vi "Eigenschaften laden.vi"(8 "error in (no error)":errorcluster caption="Fehler (Eingang)", 11 "TDMS-Datei":refnum<k34>) -> (0 "error out":errorcluster caption="Fehler (Ausgang)", 1 "Datentypen":string[](array[string]), 2 "Namen":string[](array[string]), 3 "TDMS-Datei (Ausgang)":refnum<k34>, 4 "Eigenschaften":T1)   [LabVIEW 2020, in "Anlagenuebersicht.lvlib" / "VisBx Anzeige.lvlib" / "TDMS laden.lvlib"]
doc: "Liest aus einer bereits geöffneten TDMS-Datei für die Visualisierungs-Anwendung \"VisBx Anzeige\":\n\nNamen:\nNamen aller Prozessvariablen, die Grundlage für die TDMS-Datei waren.\n\nDatentypen:\nDatentypen aller Prozessvariablen.\n\nEigenschaften:\nCluster mit den Elementen\n Größe: Bildgröße der Visualisierung (Width, Height)\n URL: String mit URL der XML-Umgebungsvariablen für die Prozesskopplung\n Raster: letztes Rastermaß (wird nur für Editor gebraucht)\n Hintergrund: Hintergrundfarbe der Visualisierung (nur für Editor)."
uses:
  TDMS laden.lvlib
  TDMS-Eigenschaften.ctl
  <vilib>/Utility/miscctls.llb/LVBoundsTypeDef.ctl
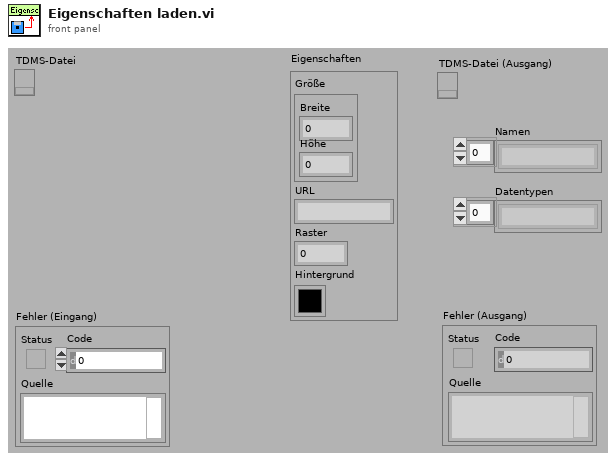
[diagram p1: front panel]
types:
  T1 = typedef "Anlagenuebersicht.lvlib/VisBx Anzeige.lvlib/TDMS laden.lvlib/TDMS-Eigenschaften.ctl" = cluster{"Größe":T2, "URL":string, "Raster":i16, "Hintergrund":u32}
  T2 = typedef "LVBoundsTypeDef.ctl" = cluster{"Width":u32, "Height":u32}
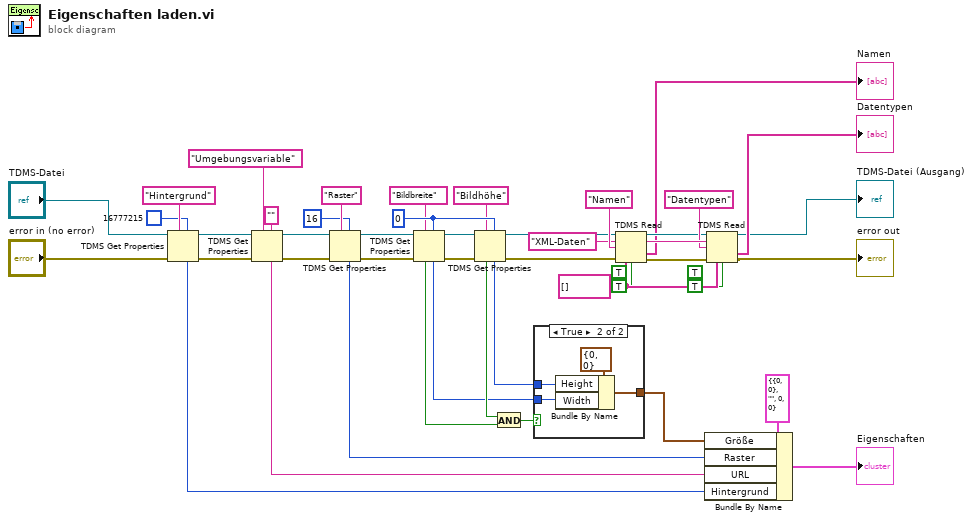
[diagram p0: block diagram]
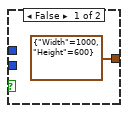
[diagram p2: hidden frame]
diagram:
  (unwired) TRUE ("Kanalreihenfolge von Datei beibehalten? (F)")
  (unwired) TRUE ("Kanalreihenfolge von Datei beibehalten? (F)")
  w27 = u32 0 ("Height")
  w38 = string[] [] ("Typen (ohne Cluster)")
  n1 = TDMS Get Properties(5:u32 16777215, 7:"Hintergrund" ("Eigenschaftsname"), 8:"error in (no error)", 11:"TDMS-Datei") -> (0:w8:errorcluster, 3:w10:refnum<k34>, 4:w5:u32)  [unwired: 5 out]
  n2 = TDMS Get Properties(5:"", 7:"Umgebungsvariable", 8:w8, 11:w10) -> (0:w20:errorcluster, 3:w22:refnum<k34>, 4:w13:string)  [unwired: 5 out]
  n3 = TDMS Get Properties(5:i16 16 ("Height"), 7:"Raster" ("Eigenschaftsname"), 8:w20, 11:w22) -> (0:w19:errorcluster, 3:w21:refnum<k34>, 4:w14:i16)  [unwired: 5 out]
  n4 = TDMS Get Properties(5:w27, 7:"Bildbreite" ("Eigenschaftsname"), 8:w19, 11:w21) -> (0:w29:errorcluster, 3:w28:refnum<k34>, 4:w31:u32, 6:w34:bool)  [unwired: 4 out]
  n5 = TDMS Get Properties(5:w27, 7:"Bildhöhe" ("Eigenschaftsname"), 8:w29, 11:w28) -> (0:w17:errorcluster, 3:w18:refnum<k34>, 4:w30:u32, 6:w33:bool)  [unwired: 4 out]
  n6 = And(x=w33, y=w34) -> (x .and. y?=w32:bool)
  n7 = case shown="True" w32 {
    tunnel: [T2 {"Width"=1000, "Height"=600} ("Darstellungsbereich") w49] -> w15
    tunnel: w30 -> [_ w48]
    tunnel: w31 -> [_ w47]
    frame False {
    }
    frame True {
      n8 = Bundle By Name(cluster=T2 {"Width"=0, "Height"=0} ("Darstellungsbereich"), "Height"=w48, "Width"=w47) -> (w49:T2)
    }
  }
  n9 = TDMS Read(0:w18, 5:"XML-Daten" ("Gruppenname (Eingang, Unbenannt)"), 7:"Namen", 11:w17, 12:w38, 13:TRUE ("Kanalreihenfolge von Datei beibehalten? (F)")) -> (4:w39:refnum<k34>, 6:w45:string, 10:→"Namen":string[], 15:w4:errorcluster)  [unwired: 2 in, 2 out]
  n10 = Bundle By Name(cluster=T1 {"Größe"={"Width"=0, "Height"=0}, "URL"="", "Raster"=0, "Hintergrund"=0} ("Eigenschaften"), "Größe"=w15, "Raster"=w14, "URL"=w13, "Hintergrund"=w5) -> (→"Eigenschaften":T1)
  n11 = TDMS Read(0:w39, 5:w45, 7:"Datentypen", 11:w4, 12:w38, 13:TRUE ("Kanalreihenfolge von Datei beibehalten? (F)")) -> (4:→"TDMS-Datei (Ausgang)":refnum<k34>, 10:→"Datentypen":string[], 15:→"error out":errorcluster)  [unwired: 2 in, 3 out]
